vi "Find eTDS COM Port.vi"() -> (1 "USB port":refnum<visa-resource-name>, 2 "None/Multiple Device(s)?":bool)   [LabVIEW 2013]
uses:
  <vilib>/Utility/error.llb/whitespace.ctl
panel:
  out "COM PORTS":refnum<visa-resource-name>[](array[refnum])
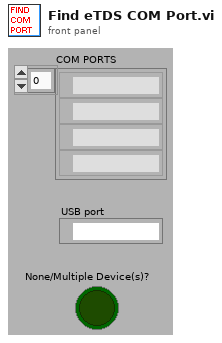
[diagram p1: front panel]
types:
  T1 = typedef "whitespace.ctl" = u16
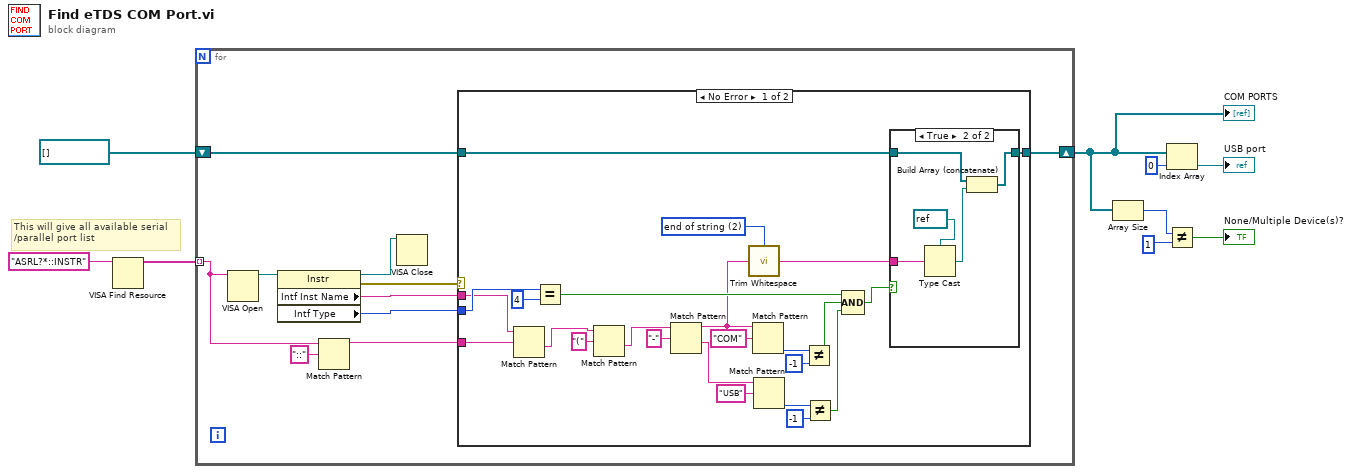
[diagram p0: block diagram]
diagram:
  # "This will give all available serial\n/parallel port list"
  n1 = VISA Find Resource(11:"ASRL?*::INSTR" ("expression (\"\")")) -> (3:w7:string[])  [unwired: 1 in, 3 out]
  n2 = for {
    shift-right: [w14] -> w3
    shift-left: refnum<visa-resource-name>[] [] -> [w15]
    tunnel: w7 -> [w12] mode=indexing
    n3 = VISA Open(VISA resource name=w12) -> (VISA resource name=w11:refnum<visa-resource-name>)  [unwired: 1 in, 4 out]
    n4 = property class="Instr"(reference=w11) -> (reference out=w10:refnum<visa-resource-name>, error out=w19:errorcluster, "Intf Inst Name"=w18:string, "Intf Type"=w17:u16)  [unwired: 1 in]
    n5 = Match Pattern(string=w12, regular expression="::") -> (before substring=w13:string)  [unwired: 4 out]
    n6 = VISA Close(VISA resource name=w10) -> ()  [unwired: 1 in, 1 out]
    n7 = case shown="No Error" w19 {
      tunnel: w18 -> [w21 _]
      tunnel: w17 -> [w36 _]
      tunnel: w13 -> [w41 _]
      tunnel: w15 -> [w31 w50]
      tunnel: [w30 w50] -> w14
      frame No Error {
        w29 = T1 2 items=["both", "start of string", "end of string"] ("location (both)")
        n8 = Match Pattern(string=w21, regular expression=w41) -> (after substring=w40:string)  [unwired: 4 out]
        n9 = Equal?(x=w36, y=u16 4) -> (x = y?=w34:bool)
        n10 = Match Pattern(string=w40, regular expression="(") -> (after substring=w27:string)  [unwired: 4 out]
        n11 = Match Pattern(string=w27, regular expression="-") -> (before substring=w20:string, after substring=w23:string)  [unwired: 3 out]
        n12 = call <vilib>:"Trim Whitespace.vi"("string"=w20, "location (both)"=w29) -> ("trimmed string"=w28:string)
        n13 = Match Pattern(string=w20, regular expression="COM") -> (offset past match=w38:i32)  [unwired: 4 out]
        n14 = Match Pattern(string=w23, regular expression="USB") -> (offset past match=w25:i32)  [unwired: 4 out]
        n15 = Not Equal?(x=w38, y=-1) -> (x != y?=w33:bool)
        n16 = Not Equal?(x=w25, y=-1) -> (x != y?=w22:bool)
        n17 = Compound Arithmetic op=AND(w34, w33, w22) -> (w32:bool)
        n18 = case shown="True" w32 {
          tunnel: w28 -> [_ w48]
          tunnel: w31 -> [w44 w46]
          tunnel: [w44 w45] -> w30
          frame False {
          }
          frame True {
            n19 = Type Cast(type=refnum<visa-resource-name> refnum ("*(type *) &x"), x=w48) -> (*(type *) &x=w47:refnum<visa-resource-name>)
            n20 = Build Array (concatenate)(w46, w47) -> (w45:refnum<visa-resource-name>[])
          }
        }
      }
      frame Error {
      }
    }
  }
  "COM PORTS" <- w3
  n21 = Array Size(array=w3) -> (size(s)=w6:i32)
  n22 = Index Array(array=w3, index=0) -> (element=→"USB port":refnum<visa-resource-name>)
  n23 = Not Equal?(x=w6, y=1) -> (x != y?=→"None/Multiple Device(s)?":bool)
